vi "Write Boolean.vi"(10 "Boolean":bool, 11 "Event in":refnum<class "Event Boolean.lvclass">) -> (3 "Event out":refnum<class "Event Boolean.lvclass">)   [LabVIEW 2016, in "Event Actors.lvlib" / "Event Boolean.lvclass"]
uses:
  Event Boolean.lvclass
  Event Boolean.lvclass/Event Boolean.ctl
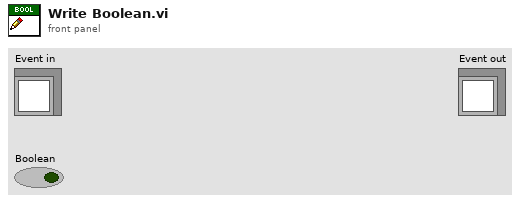
[diagram p1: front panel]
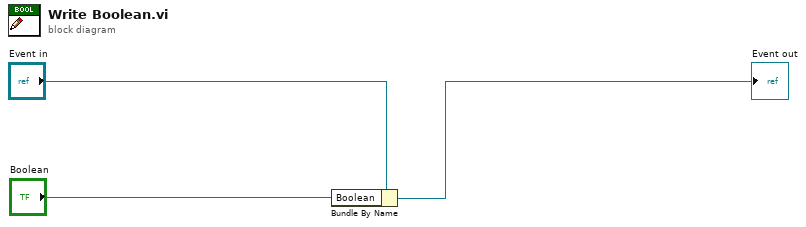
[diagram p0: block diagram]
diagram:
  n1 = Bundle By Name(cluster="Event in", "Boolean"="Boolean") -> (→"Event out":refnum<class "Event Boolean.lvclass">)
